vi "http check to keep listening.vi"(11 "application request in":T1) -> (2 "stop listening":bool, 3 "application request out":T1)   [LabVIEW 2016, in "Basic HTTP server.lvclass"]
uses:
  Basic HTTP server.lvclass
  http request.ctl
  http method.ctl
  HTTP headers/http header data.ctl
  HTTP headers/http headers.lvlib
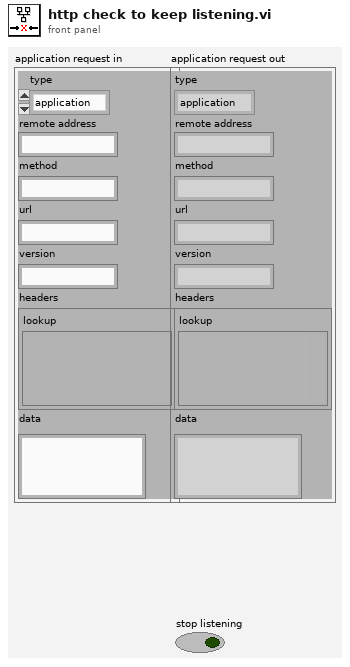
[diagram p1: front panel]
types:
  T1 = typedef "Basic HTTP server.lvclass/http request.ctl" = cluster{"type":T2, "remote address":string, "method":string, "url":string, "version":string, "headers":T3, "data":string}
  T2 = typedef "Basic HTTP server.lvclass/http method.ctl" = enum16{"application", "error", "upgrade", "expect"}
  T3 = typedef "http headers.lvlib/http header data.ctl" = cluster{"lookup":variant}
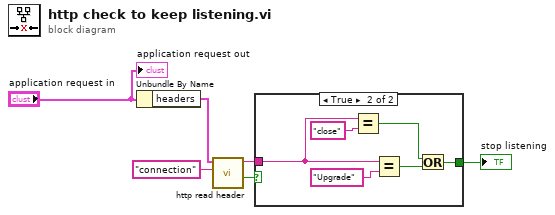
[diagram p0: block diagram]
diagram:
  n1 = Unbundle By Name("application request in") -> ("headers"=w3:T3)
  n2 = call "http read header.vi"("header field name"="connection" ("name"), "headers"=w3) -> ("found"=w5:bool, "value"=w1:string)  [unwired: 8 in]
  n3 = case shown="True" w5 {
    tunnel: w1 -> [_ w12]
    tunnel: [_ w11] -> w6
    frame False {
    }
    frame True {
      n4 = Equal?(x=w12, y="close" ("name")) -> (x = y?=w10:bool)
      n5 = Equal?(x=w12, y="Upgrade" ("name")) -> (x = y?=w7:bool)
      n6 = Or(x=w10, y=w7) -> (x .or. y?=w11:bool)
    }
  }
  "stop listening" <- w6
  "application request out" <- "application request in"
